vi "CC_Fpga.vi"() -> ()   [LabVIEW 2019]
uses:
  <vilib>/rvi/Emulation/niFpgaGetClockAttributes.vi
  <vilib>/rvi/Emulation/niFpgaSctlEmulationGetInTimedLoop.vi
  <vilib>/rvi/Emulation/niFpgaEmulationReportErrorSimple.vi
  <vilib>/rvi/eio/common/nirviEmuTemplateMethod_errors.vi
  <vilib>/rvi/Emulation/niFpgaCriticalErrorInLSC.vi
  <vilib>/eio/EIONode/EIONode.xnode
  <vilib>/rvi/Arithmetic/AddSubMult/XNode/nirviSatArithmetic.xnode
panel:
  out "current control o/p":sgl
  in  "Proportional Gain":sgl
  out "raw current":sgl
  in  "Position Reset 2":bool
  in  "Velocity Interval (uSec) 2 motor side":u32=1000
  out "Position (Counts) motor side":i32(graph)
  out "Acceleration (Counts/Interval) 2 motor side":i32
  out "Velocity (Counts/Interval) 2 motor side":i32
  out "Loop time (position) 2 motor side":u32
  out "motor direction":bool
  out "Loop time(current)":u32
  in  "Position Reset":bool
  in  "Velocity Interval (uSec) joint side":u32=1000
  out "Position (Counts) joint side":i32(graph)
  out "Acceleration (Counts/Interval) joint side":i32
  out "Velocity (Counts/Interval) joint side":i32
  out "Loop time (position) 1 joint side":u32
  in  "current offset":sgl
  in  "setpoint":sgl
  out "error\nerror":sgl(knob) scale=-100.0..100.0
  out "filtered current":sgl(graph)
  out "Raw voltage data":sgl(graph)
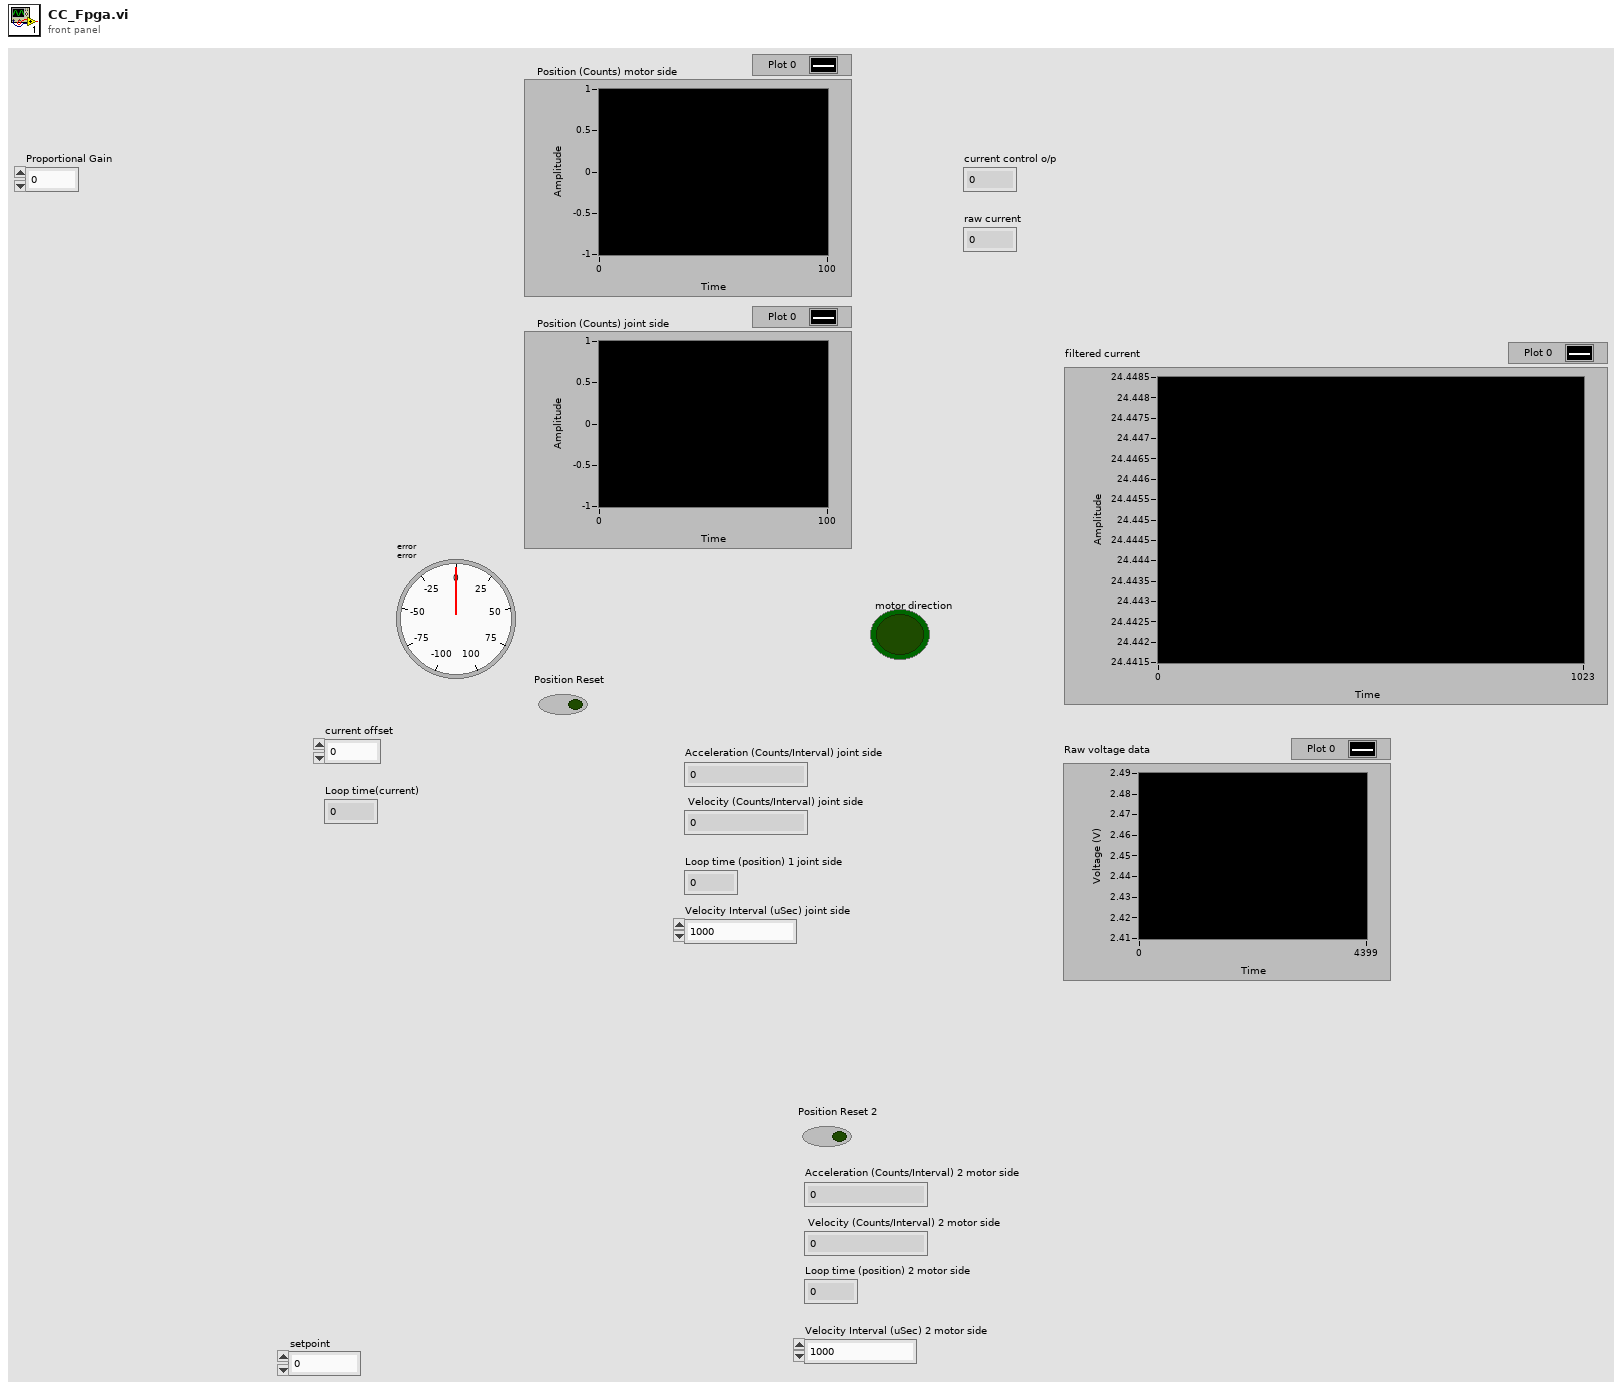
[diagram p1: front panel]
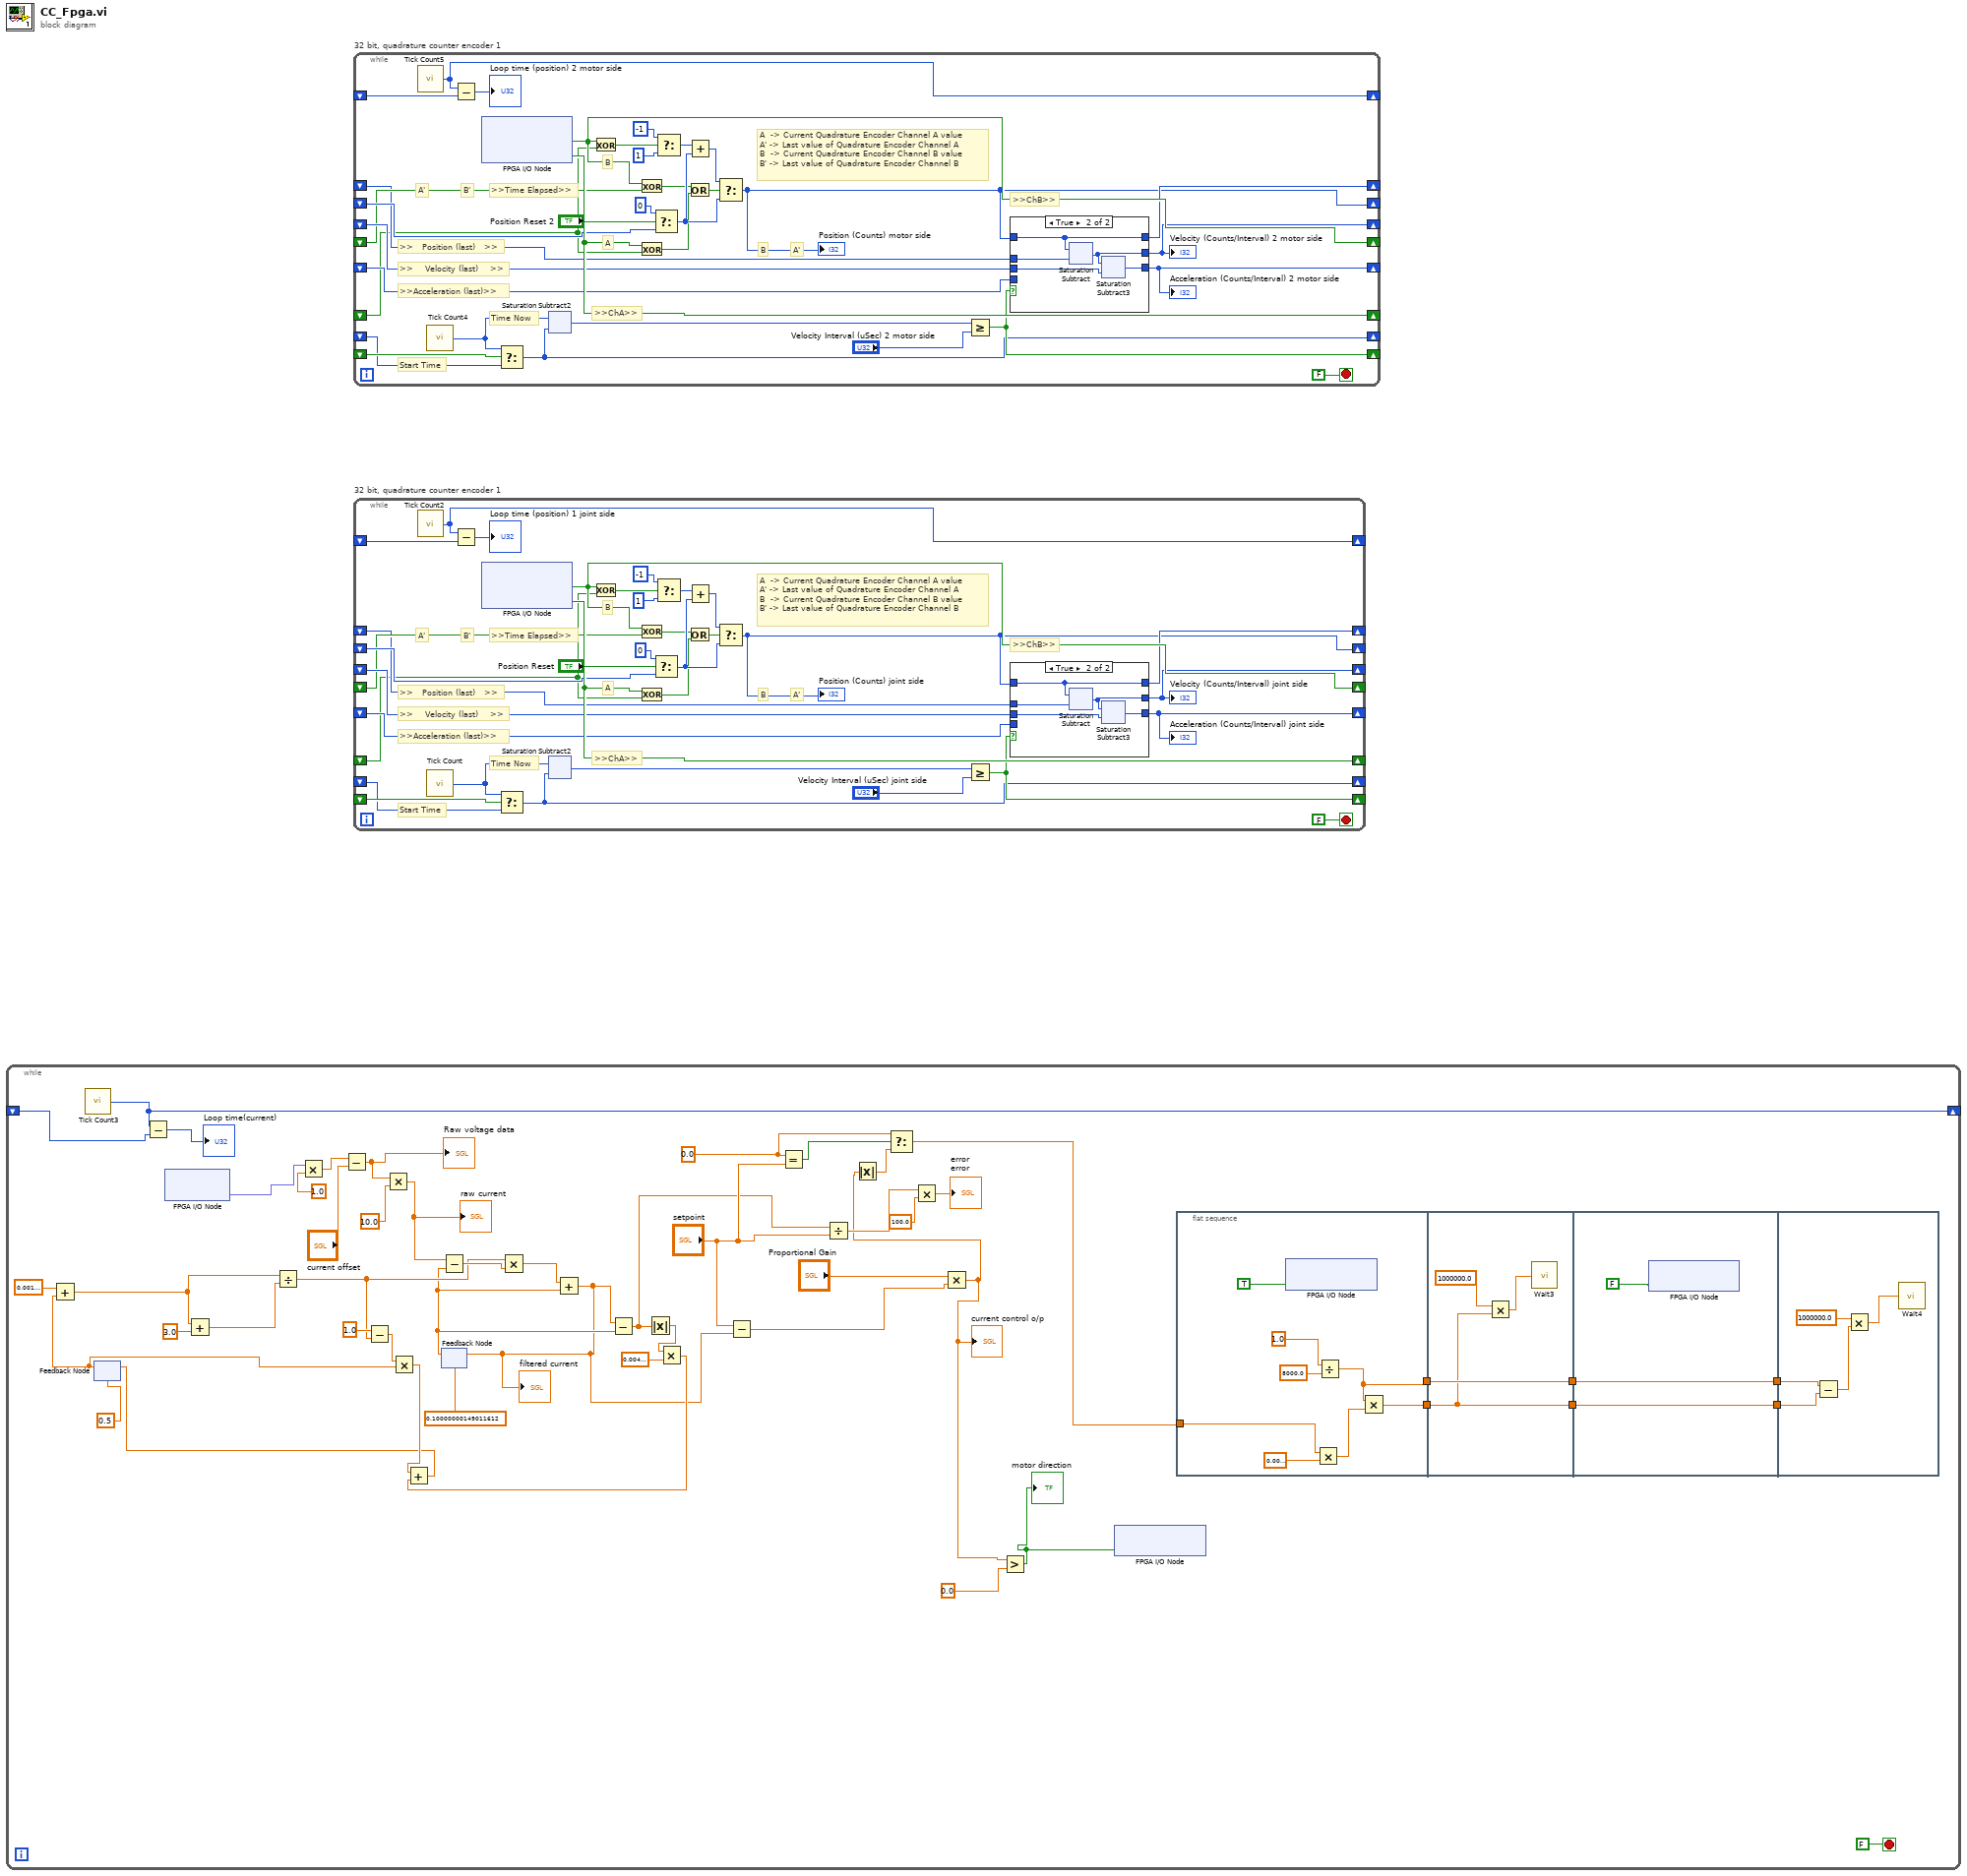
[diagram p0: block diagram]
diagram:
  n1 = while {
    shift-right: [w12] -> _
    shift-left: _ -> [w11]
    stop <- FALSE stop-if-true
    w18 = sgl 0.0 ("x")
    n2 = call "Tick Count3"() -> ("Tick Count(Ticks)"=w12:u32)
    n3 = feedback #1(sgl 0.5) -> (w35:sgl)
    n4 = Add(x=sgl 0.001, y=w35) -> (x+y=w44:sgl)
    n5 = Subtract(x=w12, y=w11) -> (x-y=→"Loop time(current)":u32)
    n6 = xnode "FPGA I/O Node"() -> ("AI0"=w48:fxp<+/-,24,5>)  [unwired: 1 in, 1 out]
    n7 = Add(x=w44, y=sgl 3.0) -> (x+y=w43:sgl)
    n8 = Divide(x=w44, y=w43) -> (x/y=w37:sgl)
    n9 = Multiply(x=w48, y=sgl 1.0) -> (x*y=w49:sgl)
    n10 = Subtract(x=w49, y="current offset") -> (x-y=w47:sgl)
    "Raw voltage data" <- w47
    n11 = Subtract(x=sgl 1.0, y=w37) -> (x-y=w36:sgl)
    n12 = Multiply(x=w47, y=sgl 10.0) -> (x*y=w42:sgl)
    "raw current" <- w42
    n13 = Multiply(x=w36, y=w35) -> (x*y=w34:sgl)
    n14 = feedback #2(sgl 0.1) -> (w33:sgl)
    n15 = Subtract(x=w42, y=w33) -> (x-y=w40:sgl)
    n16 = Multiply(x=w37, y=w40) -> (x*y=w39:sgl)
    n17 = Add(x=w39, y=w33) -> (x+y=w1:sgl)
    "filtered current" <- w1
    n18 = feedback-in #2(w1) -> ()
    n19 = Subtract(x=w1, y=w33) -> (x-y=w8:sgl)
    n20 = Absolute Value(x=w8) -> (abs(x)=w32:sgl)
    n21 = Multiply(x=w32, y=sgl 0.005) -> (x*y=w2:sgl)
    n22 = Add(x=w34, y=w2) -> (x+y=w31:sgl)
    n23 = feedback-in #1(w31) -> ()
    n24 = Subtract(x="setpoint", y=w1) -> (x-y=w7:sgl)
    n25 = Equal?(x=w18, y="setpoint") -> (x = y?=w17:bool)
    n26 = Divide(x=w8, y="setpoint") -> (x/y=w30:sgl)
    n27 = Multiply(x=w30, y=sgl 100.0) -> (x*y=→"error\nerror":sgl)
    n28 = Multiply(x="Proportional Gain", y=w7) -> (x*y=w4:sgl)
    "current control o/p" <- w4
    n29 = Absolute Value(x=w4) -> (abs(x)=w16:sgl)
    n30 = Select(t=w18, s=w17, f=w16) -> (s? t:f=w15:sgl)
    n31 = Greater?(x=w4, y=sgl 0.0) -> (0:w3:bool)
    "motor direction" <- w3
    n32 = xnode "FPGA I/O Node"("RMC/DIO51"=w3) -> ()  [unwired: 1 in, 1 out]
    n33 = flat-sequence {
      tunnel: [w55] -> w24
      tunnel: [w54] -> w23
      tunnel: w15 -> [w51]
      tunnel: w24 -> [w61]
      tunnel: w23 -> [w62]
      tunnel: [w61] -> w22
      tunnel: [w62] -> w21
      tunnel: w22 -> [w65]
      tunnel: w21 -> [w64]
      tunnel: [w65] -> w20
      tunnel: [w64] -> w19
      tunnel: w20 -> [w69]
      tunnel: w19 -> [w70]
      frame #0 {
        n34 = xnode "FPGA I/O Node"("RMC/DIO49"=TRUE) -> ()  [unwired: 1 in, 1 out]
        n35 = Multiply(x=w51, y=sgl 0.01) -> (x*y=w56:sgl)
        n36 = Divide(x=sgl 1.0, y=sgl 8000.0) -> (x/y=w54:sgl)
        n37 = Multiply(x=w54, y=w56) -> (x*y=w55:sgl)
      }
      frame #1 {
        n38 = Multiply(x=sgl 1000000.0, y=w61) -> (x*y=w60:sgl)
        n39 = call "Wait3"("Count(uSec)"=w60) -> ()  [unwired: 1 out]
      }
      frame #2 {
        n40 = xnode "FPGA I/O Node"("RMC/DIO49"=FALSE) -> ()  [unwired: 1 in, 1 out]
      }
      frame #3 {
        n41 = Subtract(x=w70, y=w69) -> (x-y=w68:sgl)
        n42 = Multiply(x=sgl 1000000.0, y=w68) -> (x*y=w67:sgl)
        n43 = call "Wait4"("Count(uSec)"=w67) -> ()  [unwired: 1 out]
      }
    }
  }
  n44 = while "32 bit, quadrature counter encoder 1" {
    shift-right: [w94] -> _
    shift-left: _ -> [w81]
    shift-right: [w77] -> _
    shift-left: _ -> [w91]
    shift-right: [w93] -> _
    shift-left: _ -> [w71]
    shift-right: [w87] -> _
    shift-left: _ -> [w90]
    shift-right: [w83] -> _
    shift-left: _ -> [w88]
    shift-right: [w78] -> _
    shift-left: _ -> [w76]
    shift-right: [w79] -> _
    shift-left: _ -> [w85]
    shift-right: [w80] -> _
    shift-left: _ -> [w82]
    shift-right: [w73] -> _
    shift-left: _ -> [w75]
    stop <- FALSE stop-if-true
    # "A  -> Current Quadrature Encoder Channel A value\nA' -> Last value of Quadrature Encoder Channel A\nB  -> Current Quadrature Encoder Channel B value\nB' -> Last value of Quadrature Encoder Channel B"
    # ">>Acceleration (last)>>"
    # "Start Time"
    # "A'"
    # "B"
    # "A'"
    # "A"
    # "B'"
    # "B"
    # ">>ChB>>"
    # ">>ChA>>"
    # ">>    Velocity (last)    >>"
    # ">>   Position (last)   >>"
    # "Time Now"
    # ">>Time Elapsed>>"
    n45 = call "Tick Count5"() -> ("Tick Count(Ticks)"=w73:u32)
    n46 = call "Tick Count4"() -> ("Tick Count(uSec)"=w84:u32)
    n47 = Subtract(x=w73, y=w75) -> (x-y=→"Loop time (position) 2 motor side":u32)
    n48 = xnode "FPGA I/O Node"() -> ("RMC/DIO59"=w94:bool, "RMC/DIO57"=w93:bool)  [unwired: 2 in, 2 out]
    n49 = Select(t=w84, s=w90, f=w88) -> (s? t:f=w83:u32)
    n50 = xnode ("Saturation Subtract2")("x"=w84, "y"=w83) -> ("x-y"=w86:u32)
    n51 = Exclusive Or(1:w71, 2:w94) -> (0:w95:bool)
    n52 = Exclusive Or(1:w81, 2:w94) -> (0:w96:bool)
    n53 = Exclusive Or(1:w71, 2:w93) -> (0:w97:bool)
    n54 = Select(t=0 ("32 bit"), s="Position Reset 2", f=w91) -> (s? t:f=w102:i32)
    n55 = Select(t=-1 ("32 bit"), s=w95, f=1 ("32 bit")) -> (s? t:f=w100:i32)
    n56 = Add(x=w100, y=w102) -> (x+y=w104:i32)
    n57 = Or(x=w96, y=w97) -> (x .or. y?=w92:bool)
    n58 = Select(t=w104, s=w92, f=w102) -> (s? t:f=w77:i32)
    "Position (Counts) motor side" <- w77
    n59 = Greater Or Equal?(x=w86, y="Velocity Interval (uSec) 2 motor side") -> (x >= y?=w87:bool)
    n60 = case shown="True" w87 {
      tunnel: w77 -> [_ w118]
      tunnel: w76 -> [w115 w122]
      tunnel: [w117 w121] -> w79
      tunnel: w85 -> [w117 w120]
      tunnel: [w116 w119] -> w80
      tunnel: w82 -> [w116 _]
      tunnel: [w115 w118] -> w78
      frame False {
      }
      frame True {
        n61 = xnode ("Saturation Subtract")("x"=w118, "y"=w122) -> ("x-y"=w121:i32)
        n62 = xnode ("Saturation Subtract3")("x"=w121, "y"=w120) -> ("x-y"=w119:i32)
      }
    }
    "Acceleration (Counts/Interval) 2 motor side" <- w80
    "Velocity (Counts/Interval) 2 motor side" <- w79
  }
  n63 = while "32 bit, quadrature counter encoder 1" {
    shift-right: [w182] -> _
    shift-left: _ -> [w169]
    shift-right: [w165] -> _
    shift-left: _ -> [w179]
    shift-right: [w181] -> _
    shift-left: _ -> [w159]
    shift-right: [w175] -> _
    shift-left: _ -> [w178]
    shift-right: [w171] -> _
    shift-left: _ -> [w176]
    shift-right: [w166] -> _
    shift-left: _ -> [w164]
    shift-right: [w167] -> _
    shift-left: _ -> [w173]
    shift-right: [w168] -> _
    shift-left: _ -> [w170]
    shift-right: [w161] -> _
    shift-left: _ -> [w163]
    stop <- FALSE stop-if-true
    # "A  -> Current Quadrature Encoder Channel A value\nA' -> Last value of Quadrature Encoder Channel A\nB  -> Current Quadrature Encoder Channel B value\nB' -> Last value of Quadrature Encoder Channel B"
    # ">>Acceleration (last)>>"
    # "Start Time"
    # "A'"
    # "B"
    # "A'"
    # "A"
    # "B'"
    # "B"
    # ">>ChB>>"
    # ">>ChA>>"
    # ">>    Velocity (last)    >>"
    # ">>   Position (last)   >>"
    # "Time Now"
    # ">>Time Elapsed>>"
    n64 = call "Tick Count2"() -> ("Tick Count(Ticks)"=w161:u32)
    n65 = call "Tick Count"() -> ("Tick Count(uSec)"=w172:u32)
    n66 = Subtract(x=w161, y=w163) -> (x-y=→"Loop time (position) 1 joint side":u32)
    n67 = xnode "FPGA I/O Node"() -> ("RMC/DIO55"=w182:bool, "RMC/DIO54"=w181:bool)  [unwired: 2 in, 2 out]
    n68 = Select(t=w172, s=w178, f=w176) -> (s? t:f=w171:u32)
    n69 = xnode ("Saturation Subtract2")("x"=w172, "y"=w171) -> ("x-y"=w174:u32)
    n70 = Exclusive Or(1:w159, 2:w182) -> (0:w183:bool)
    n71 = Exclusive Or(1:w169, 2:w182) -> (0:w184:bool)
    n72 = Exclusive Or(1:w159, 2:w181) -> (0:w185:bool)
    n73 = Select(t=0 ("32 bit"), s="Position Reset", f=w179) -> (s? t:f=w190:i32)
    n74 = Select(t=-1 ("32 bit"), s=w183, f=1 ("32 bit")) -> (s? t:f=w188:i32)
    n75 = Add(x=w188, y=w190) -> (x+y=w192:i32)
    n76 = Or(x=w184, y=w185) -> (x .or. y?=w180:bool)
    n77 = Select(t=w192, s=w180, f=w190) -> (s? t:f=w165:i32)
    "Position (Counts) joint side" <- w165
    n78 = Greater Or Equal?(x=w174, y="Velocity Interval (uSec) joint side") -> (x >= y?=w175:bool)
    n79 = case shown="True" w175 {
      tunnel: w165 -> [_ w206]
      tunnel: w164 -> [w203 w210]
      tunnel: [w205 w209] -> w167
      tunnel: w173 -> [w205 w208]
      tunnel: [w204 w207] -> w168
      tunnel: w170 -> [w204 _]
      tunnel: [w203 w206] -> w166
      frame False {
      }
      frame True {
        n80 = xnode ("Saturation Subtract")("x"=w206, "y"=w210) -> ("x-y"=w209:i32)
        n81 = xnode ("Saturation Subtract3")("x"=w209, "y"=w208) -> ("x-y"=w207:i32)
      }
    }
    "Acceleration (Counts/Interval) joint side" <- w168
    "Velocity (Counts/Interval) joint side" <- w167
  }
